vi "WPI_CameraDraw Text to Image.vi"(9 "BG Color":u32(colorbox)=5789784, 10 "Text":string, 11 "Refnum in":T1) -> (3 "Refnum out":T1)   [LabVIEW 2017]
uses:
  <vilib>/vision/Image Controls.llb/IMAQ Image.ctl
  <vilib>/vision/NI_Vision_Development_Module.lvlib
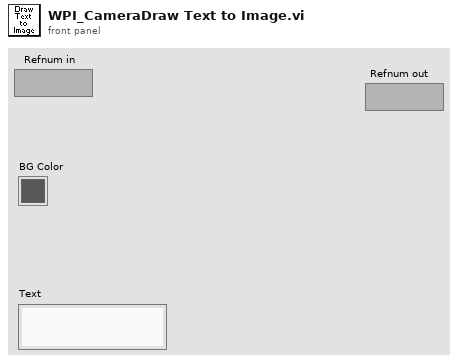
[diagram p1: front panel]
types:
  T1 = typedef "IMAQ Image.ctl" = refnum<image>
  T2 = cluster{"Desired Font (Application)":enum16{"User-specified Font", "Application Font", "System Font", "Dialog Font"}, "[User-specified Font]":cluster{"Font Name":string, "Size":i16, "Strikeout?":bool, "Italic?":bool, "Underline?":bool, "Outline?":bool, "Shadow?":bool, "Bold?":bool, "Rotation Angle":dbl}, "Horizontal Alignment":i16, "Vertical Alignment":i16}
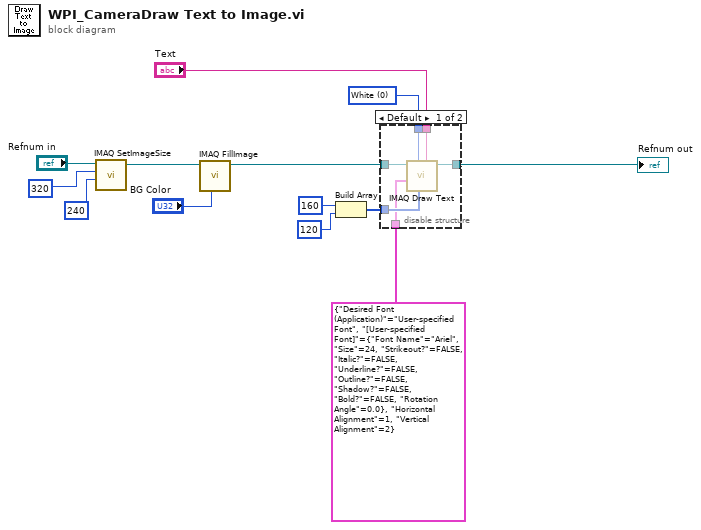
[diagram p0: block diagram]
diagram:
  w10 = 0 items=["White", "Black", "Inverted", "Black on White", "White on Black"] ("Color")
  n1 = call "IMAQ SetImageSize"("Y Resolution"=240, "X Resolution"=320, "Image"="Refnum in") -> ("Image Out"=w6:T1)  [unwired: 2 in, 1 out]
  n2 = call "IMAQ FillImage"("Color Pixel Value"="BG Color", "Image"=w6) -> ("Image Out"=w8:T1)  [unwired: 8 in, 1 out]
  n3 = Build Array(160, 120) -> (w1:i32[])
  n4 = disable-structure shown="Default" {
    disable-tunnel: [w18 w20] -> w12
    disable-tunnel: "Text" -> [w17 _]
    disable-tunnel: w10 -> [w16 _]
    disable-tunnel: T2 {"Desired Font (Application)"=enum."User-specified Font", "[User-specified Font]"={"Font Name"="Ariel", "Size"=24, "Strikeout?"=FALSE, "Italic?"=FALSE, "Underline?"=FALSE, "Outline?"=FALSE, "Shadow?"=FALSE, "Bold?"=FALSE, "Rotation Angle"=0.0}, "Horizontal Alignment"=1, "Vertical Alignment"=2} ("Font, Size & Style") -> [w14 _]
    disable-tunnel: w8 -> [w19 w20]
    disable-tunnel: w1 -> [w15 _]
    frame condition #0 {
      n5 = call "IMAQ Draw Text"("String"=w17, "Insertion Point"=w15, "Color"=w16, "Font, Size & Style"=w14, "Image Src"=w19) -> ("Image Dst Out"=w18:T1)  [unwired: 3 in, 3 out]
    }
    frame condition #1 (active) {
    }
  }
  "Refnum out" <- w12
